vi "Write Anti-aliased.vi"(5 "Anti-aliased":bool, 9 "Plot in":refnum<class "Plot.lvclass">) -> (3 "Plot out":refnum<class "Plot.lvclass">)   [LabVIEW 2014, in "Plot.lvclass"]
uses:
  Plot.lvclass
  Plot.lvclass/Plot.ctl
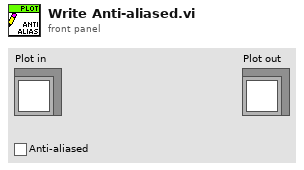
[diagram p1: front panel]
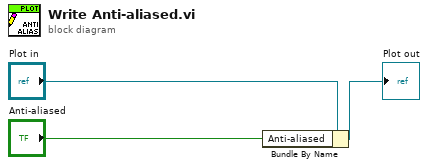
[diagram p0: block diagram]
diagram:
  n1 = Bundle By Name(cluster="Plot in", "Anti-aliased"="Anti-aliased") -> (→"Plot out":refnum<class "Plot.lvclass">)
